vi "Process.vi"(11 "TEMPLATE Actor in":refnum<class "TEMPLATE Actor.lvclass">) -> (3 "TEMPLATE Actor out":refnum<class "TEMPLATE Actor.lvclass">)   [LabVIEW 2020, in "_Template.lvlib" / "Templates.lvlib" / "TEMPLATE Actor.lvlib" / "TEMPLATE Actor.lvclass"]
uses:
  TEMPLATE Actor.lvclass
  Process Refs.ctl
  jettl/jettl/Actor/Actor/Actor.lvclass
  jettl/jettl/Msg/Msg.lvclass
  C:/git/jettl/src/jettl/jettl/Actor/Actor/Actor.lvclass
  C:/git/jettl/src/jettl/jettl/Last Ack Msg/Last Ack/Last Ack.lvclass
  C:/git/jettl/src/jettl/jettl/Teardown Msg/Teardown/Teardown.lvclass
  C:/git/jettl/src/jettl Tools/_Template/Templates/TEMPLATE Actor/TEMPLATE Actor/TEMPLATE Actor.lvclass
types:
  T1 = typedef "_Template.lvlib/Templates.lvlib/TEMPLATE Actor.lvlib/TEMPLATE Actor.lvclass/Process Refs.ctl" = cluster{"This VI":refnum<vi>}
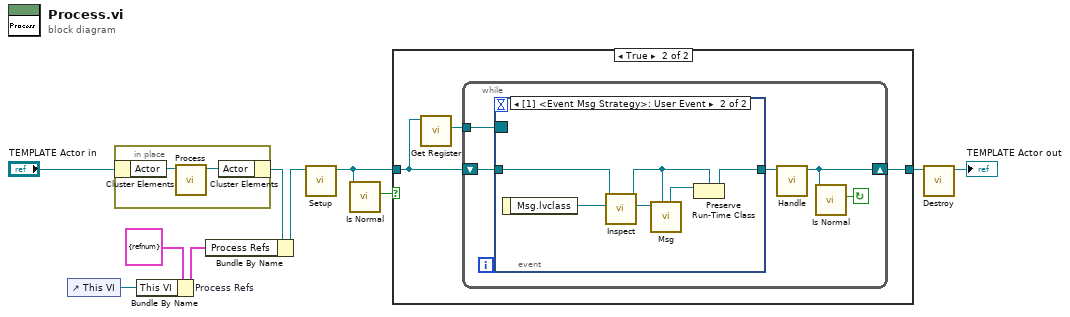
[diagram p0: block diagram]
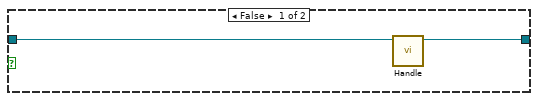
[diagram p2: hidden frame]
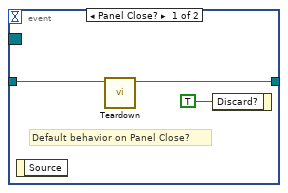
[diagram p3: hidden frame]
diagram:
  n1 = control-ref of="This VI"() -> (w6:refnum<vi>)
  n2 = in-place {
    n3 = in-place-cluster #1("TEMPLATE Actor in") -> ("Actor"=w12:refnum<class "Actor.lvclass">)
    n4 = call-dynamic "Process.vi"("Actor in"=w12) -> ("Actor out"=w11:refnum<class "Actor.lvclass">)  [unwired: 10 in]
    n5 = in-place-cluster #1("Actor"=w11) -> (w9:refnum<class "TEMPLATE Actor.lvclass">)
  }
  n6 = Bundle By Name "Process Refs"(cluster=T1 {"This VI"=refnum} ("Process Refs"), "This VI"=w6) -> (w7:T1)
  n7 = Bundle By Name(cluster=w9, "Process Refs"=w7) -> (w3:refnum<class "TEMPLATE Actor.lvclass">)
  n8 = call-dynamic "Setup.vi"("TEMPLATE Actor in"=w3) -> ("TEMPLATE Actor out"=w1:refnum<class "TEMPLATE Actor.lvclass">)  [unwired: 10 in]
  n9 = call-dynamic "Is Normal.vi"("TEMPLATE Actor in"=w1) -> ("Is Normal"=w2:bool)  [unwired: 10 in]
  n10 = case shown="True" w2 {
    tunnel: [w13 w16] -> w4
    tunnel: w1 -> [w14 w15]
    frame False {
      n11 = call-dynamic "Handle.vi"("TEMPLATE Actor in"=w14) -> ("TEMPLATE Actor out"=w13:refnum<class "TEMPLATE Actor.lvclass">)  [unwired: 10 in]
    }
    frame True {
      n12 = call-dynamic "Get Register.vi"("TEMPLATE Actor in"=w15) -> ("Register"=w17:refnum<event-registration>)  [unwired: 10 in]
      n13 = while {
        shift-right: [w19] -> w16
        shift-left: w15 -> [w21]
        tunnel: w17 -> [w22]
        stop <- w18 continue-if-true
        n14 = event shown="[1] <Event Msg Strategy>: User Event" {
          selector: w22 -> [_ _]
          dyn-events: _ -> [_ _]
          timeout: _ -> [_ _]
          tunnel: w21 -> [w24 w27]
          tunnel: [w23 w26] -> w20
          event Panel Close? {
            # "Default behavior on Panel Close?"
            n15 = event-data() -> ()  [unwired: 1 in, 1 out]
            n16 = call-dynamic "Teardown.vi"("TEMPLATE Actor in"=w24) -> ("TEMPLATE Actor out"=w23:refnum<class "TEMPLATE Actor.lvclass">)  [unwired: 10 in]
            n17 = event-data("Discard?"=TRUE) -> ()  [unwired: 1 in, 1 out]
          }
          event User Event {
            n18 = event-data() -> ("Msg.lvclass"=w28:refnum<class "Msg.lvclass">)  [unwired: 1 in]
            n19 = call-dynamic "Inspect.vi"("Msg in"=w28, "TEMPLATE Actor in"=w27) -> ("Msg out"=w29:refnum<class "Msg.lvclass">, "TEMPLATE Actor out"=w31:refnum<class "TEMPLATE Actor.lvclass">)  [unwired: 8 in]
            n20 = call-dynamic "Msg.vi"("Actor in"=w31, "Msg in"=w29) -> ("Actor out"=w30:refnum<class "Actor.lvclass">)  [unwired: 9 in]
            n21 = Preserve Run-Time Class(object in=w30, 2:w31) -> (object out=w26:refnum<class "TEMPLATE Actor.lvclass">)  [unwired: 1 in, 1 out]
          }
        }
        n22 = call-dynamic "Handle.vi"("TEMPLATE Actor in"=w20) -> ("TEMPLATE Actor out"=w19:refnum<class "TEMPLATE Actor.lvclass">)  [unwired: 10 in]
        n23 = call-dynamic "Is Normal.vi"("TEMPLATE Actor in"=w19) -> ("Is Normal"=w18:bool)  [unwired: 10 in]
      }
    }
  }
  n24 = call-dynamic "Destroy.vi"("TEMPLATE Actor in"=w4) -> ("TEMPLATE Actor out"=→"TEMPLATE Actor out":refnum<class "TEMPLATE Actor.lvclass">)  [unwired: 10 in]
